vi "Set digital mod.vi"(8 "error in":errorcluster, 9 "Digital Power?":bool, 11 "VISA resource name":refnum<visa-resource-name>) -> (0 "error out":errorcluster, 3 "VISA resource name out":refnum<visa-resource-name>)   [LabVIEW 2017]
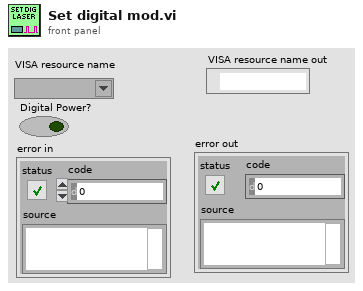
[diagram p1: front panel]
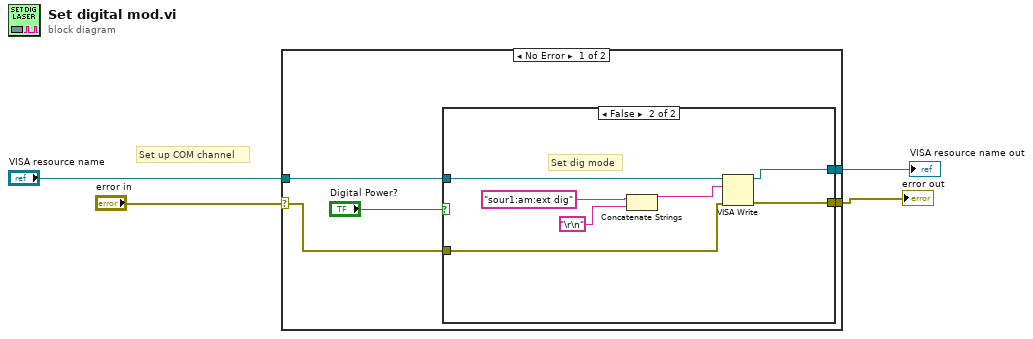
[diagram p0: block diagram]
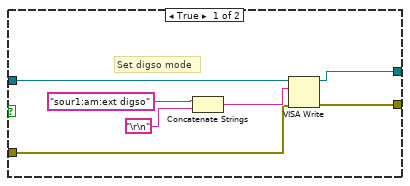
[diagram p2: hidden frame]
diagram:
  # "Set up COM channel"
  n1 = case shown="No Error" "error in" {
    selector: "error in" -> [w8 w24]
    tunnel: "VISA resource name" -> [w7 w25]
    tunnel: [w9 w24] -> w4
    tunnel: [w6 w25] -> w3
    frame No Error {
      n2 = case shown="False" "Digital Power?" {
        tunnel: [w13 w20] -> w9
        tunnel: w8 -> [w12 w19]
        tunnel: w7 -> [w11 w18]
        tunnel: [w10 w17] -> w6
        frame True {
          # "Set digso mode"
          n3 = Concatenate Strings("sour1:am:ext digso", "\r\n") -> (w14:string)
          n4 = VISA Write(VISA resource name=w11, write buffer=w14, error in (no error)=w12) -> (VISA resource name out=w10:refnum<visa-resource-name>, error out=w13:errorcluster)  [unwired: 1 out]
        }
        frame False {
          # "Set dig mode"
          n5 = Concatenate Strings("sour1:am:ext dig", "\r\n") -> (w21:string)
          n6 = VISA Write(VISA resource name=w18, write buffer=w21, error in (no error)=w19) -> (VISA resource name out=w17:refnum<visa-resource-name>, error out=w20:errorcluster)  [unwired: 1 out]
        }
      }
    }
    frame Error {
    }
  }
  "error out" <- w4
  "VISA resource name out" <- w3
